vi "Build Transfer Group.vi"(8 "error in (no error)":errorcluster, 10 "Transfer Group in":refnum<class "Transfer Group.lvclass">, 11 "Plugin Thread in":refnum<class "Plugin Thread.lvclass">) -> (0 "error out":errorcluster, 2 "Transfer Group out":refnum<class "Transfer Group.lvclass">, 3 "Plugin Thread out":refnum<class "Plugin Thread.lvclass">)   [LabVIEW 2017, in "DSF Core.lvlib" / "Plugin Thread.lvclass"]
uses:
  Thread/Plugin/Plugin Thread.lvclass
  Transfer Group/Transfer Group.lvclass
  Thread/Plugin/Plugin Thread.lvclass/Plugin Thread.ctl
  Buffer Converter/Buffer Converter.lvclass
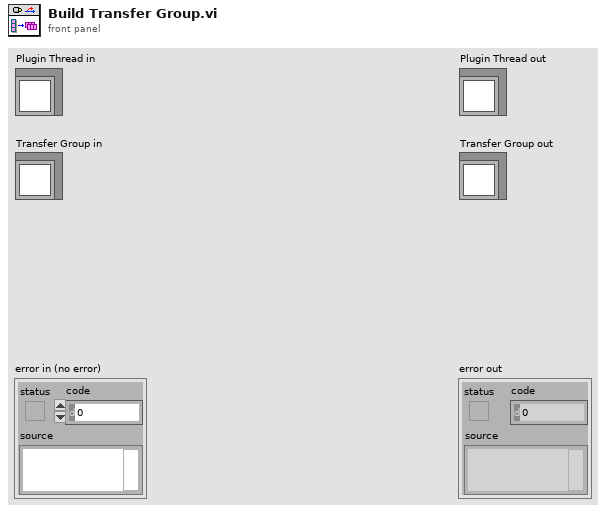
[diagram p1: front panel]
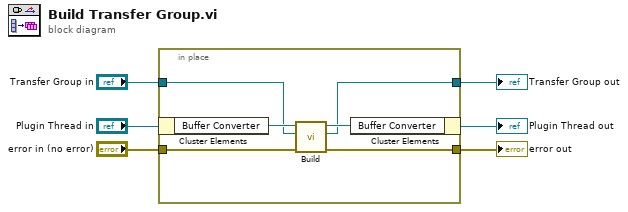
[diagram p0: block diagram]
diagram:
  n1 = in-place {
    in-place-border: "error in (no error)" -> [w10]
    in-place-border: [w9] -> w4
    in-place-border: "Transfer Group in" -> [w8]
    in-place-border: [w7] -> w1
    n2 = in-place-cluster #1("Plugin Thread in") -> ("Buffer Converter"=w12:refnum<class "Buffer Converter.lvclass">)
    n3 = call-dynamic "Build.vi"("error in (no error)"=w10, "Transfer Group in"=w8, "Buffer Converter in"=w12) -> ("error out"=w9:errorcluster, "Transfer Group out"=w7:refnum<class "Transfer Group.lvclass">, "Buffer Converter out"=w11:refnum<class "Buffer Converter.lvclass">)  [unwired: 6 in]
    n4 = in-place-cluster #1("Buffer Converter"=w11) -> (→"Plugin Thread out":refnum<class "Plugin Thread.lvclass">)
  }
  "error out" <- w4
  "Transfer Group out" <- w1
